vi "prep bdd scan.vi"(8 "tabin":string[](array[string]), 10 "Opérateur":string, 11 "SN":string) -> (0 "tabout":string[](array[string]))   [LabVIEW 2020]
uses:
  CtrldeTest/selectdata.ctl
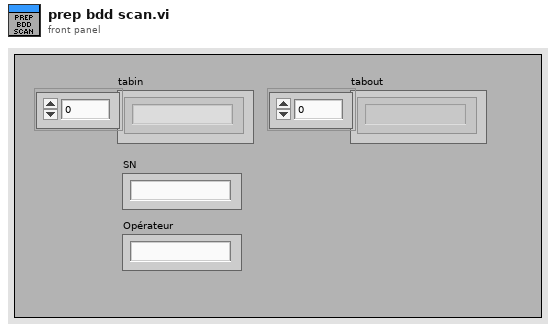
[diagram p1: front panel]
types:
  T1 = typedef "selectdata.ctl" = u16
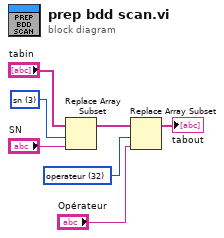
[diagram p0: block diagram]
diagram:
  w5 = T1 32 items=["id", "date", "type", "sn", "ocv", "acir", "insuP", "insuN", "TC01", "TC02", "TC11", "TC12", "TC21", "TC22", "VC01", "VC02", "VC03", "VC04", "VC11", "VC12", "VC13", "VC14", "VC21", "VC22", "VC23", "VC24", "DCIRN", "DCIRP", "inifilevers", "softvers", "imagevers", "pass", "operateur", "tpstest"] ("Menu déroulant")
  w2 = T1 3 items=["id", "date", "type", "sn", "ocv", "acir", "insuP", "insuN", "TC01", "TC02", "TC11", "TC12", "TC21", "TC22", "VC01", "VC02", "VC03", "VC04", "VC11", "VC12", "VC13", "VC14", "VC21", "VC22", "VC23", "VC24", "DCIRN", "DCIRP", "inifilevers", "softvers", "imagevers", "pass", "operateur", "tpstest"] ("Menu déroulant")
  n1 = Replace Array Subset(array="tabin", new element="SN", index=w2) -> (w4:string[])
  n2 = Replace Array Subset(array=w4, new element="Opérateur", index=w5) -> (→"tabout":string[])
